vi "Test Serialization.vi"() -> ()   [LabVIEW 2014]
uses:
  reusable/PAS/Data/Main/PAS Data.lvclass
  <vilib>/NI/AQ Character Lineator/JSON Serializer/JSON Serializer.lvclass
  <vilib>/NI/AQ Character Lineator/Serialization Common/Serial Version.ctl
  reusable/PAS/Data/Cell/PAS Cell Data.lvclass
  <vilib>/NI/AQ Character Lineator/Formatter/Path Embedding.ctl
  reusable/CRDS/Data/Cell/CRDS Cell Data.lvclass
  reusable/CRDS/Data/Main/CRDS Data.lvclass
  reusable/CRDS/Cell/extParam Ctl.ctl
  reusable/CRDS/Cell/hkParam Ctl.ctl
  <vilib>/Platform/TimedLoop/XDataNode/XDataNode.xnode
  <vilib>/Platform/TimedLoop/XDataNode/nitl_modes.ctl
  <vilib>/Platform/TimedLoop/XDataNode/XDNodeRunTimeDep.lvlib
  <vilib>/Platform/TimedLoop/XDataNode/wakeup.ctl
  <vilib>/Platform/TimedLoop/XDataNode/timing_clust.ctl
panel:
  out "x-y":u32
  out "Global Start Time":i64
  in  "Boolean":bool
  in  "Stop Button":bool
  out "error out":errorcluster
  out "length":i32
  out "String":string
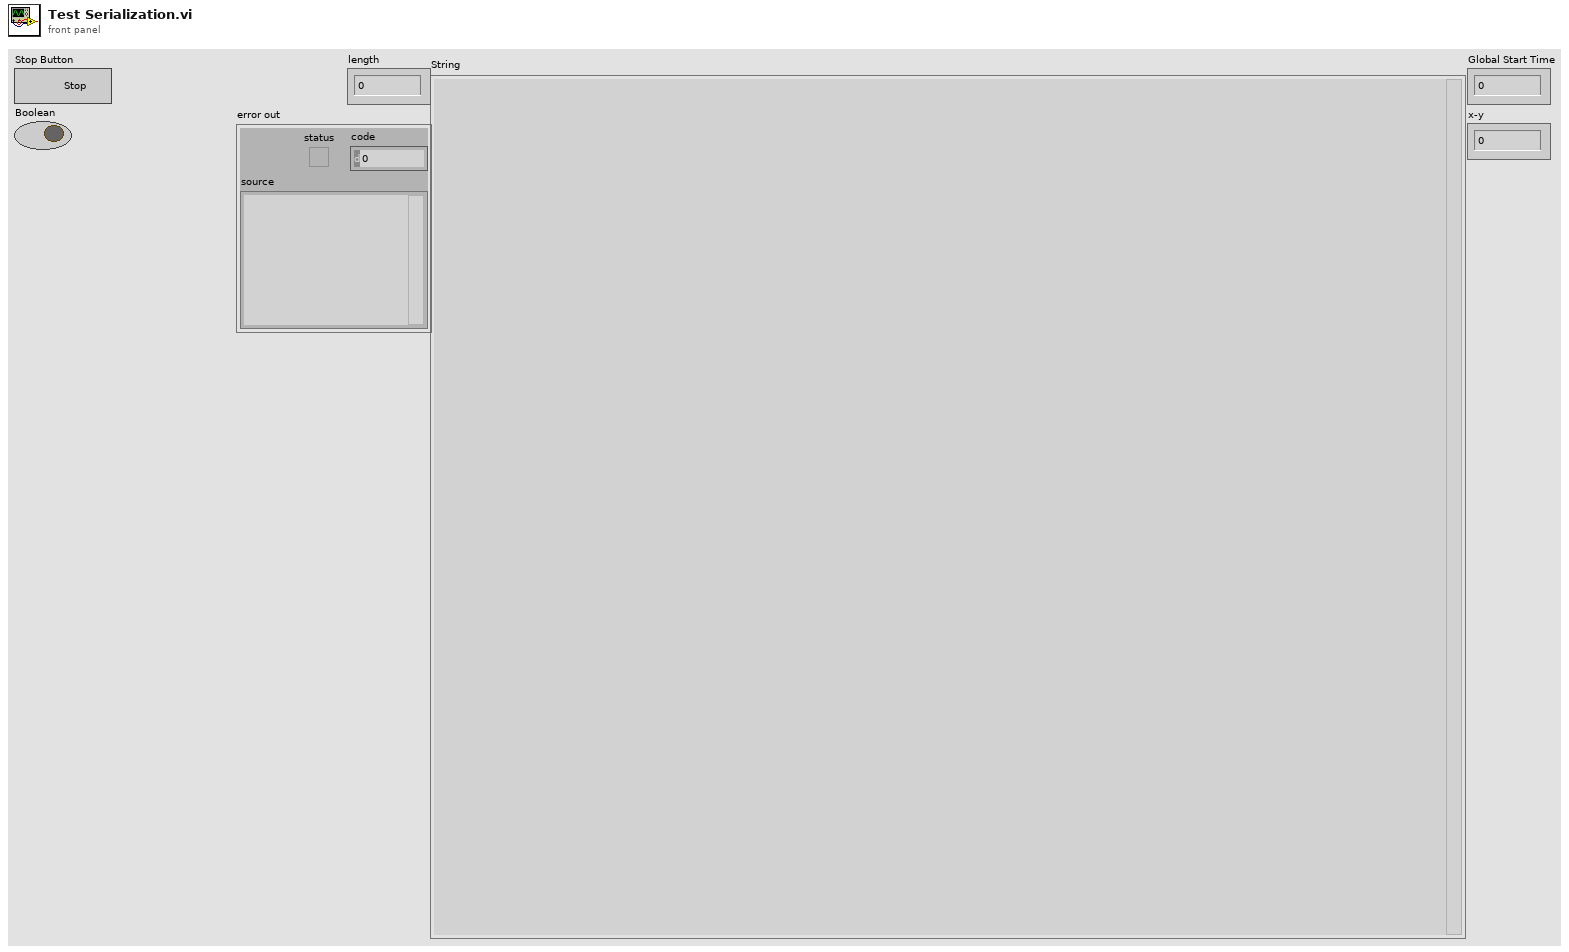
[diagram p1: front panel]
types:
  T1 = typedef "XDNodeRunTimeDep.lvlib/timing_clust.ctl" = cluster{"Expected End [f-1]":u64, "Actual End [f-1]":u64, "Finished Late? [f-1]":bool, "Expected End [i-1]":u64, "Actual End [i-1]":u64, "Finished Late? [i-1]":bool, "Expected Start [i]":u64, "Actual Start [i]":u64, "Expected Start [f]":u64, "Actual Start [f]":u64, "Source Name":string, "Structure Name":string, "Period":i64, "Deadline":i64, "Offset":i64, "Start":i64, "Priority":i32, "Timeout":i32, "Mode":T2, "Wakeup Reason":T3, "Error":errorcluster, "Source Type":string, "Secondary Source Type":string, "Global End Time":u64, "Global Start Time":u64, "Frame Duration":u64, "Iteration Duration":u64, "Assigned CPU":i32, "I/O Scan Engine Mode":u32}
  T2 = typedef "XDNodeRunTimeDep.lvlib/nitl_modes.ctl" = enum32{"No Change", "Process missed periods, maintain original phase", "Discard missed periods, maintain original phase", "Process missed periods, ignore original phase", "Discard missed periods, ignore original phase"}
  T3 = typedef "XDNodeRunTimeDep.lvlib/wakeup.ctl" = enum32{"Normal", "Aborted", "Asynchronous wakeup", "Timing source error", "Timed loop error", "Timeout"}
  T4 = typedef "Formatter.lvclass/Path Embedding.ctl" = enum16{"No paths embedded", "One path with each object", "All paths with each top object"}
  T5 = typedef "Serialization Common.lvlib/Serial Version.ctl" = cluster{"Major":u16, "Minor":u16, "Fix":u16, "Build":u16}
  T6 = typedef "CRDS Lib.lvlib/CRDS Cell Data.lvclass/hkParam Ctl.ctl" = cluster{"rhDilFac":sgl, "Q":sgl, "Tmean":sgl, "extDilFac":sgl, "rhCell":sgl, "P":sgl, "T":sgl}
  T7 = typedef "CRDS Lib.lvlib/CRDS Cell Data.lvclass/extParam Ctl.ctl" = cluster{"Tau":sgl, "Tau0cor":sgl, "ext":sgl, "extCorr":sgl, "stdevTau":sgl, "eTau":sgl, "taucorr":sgl, "Tau0":sgl, "max":sgl}
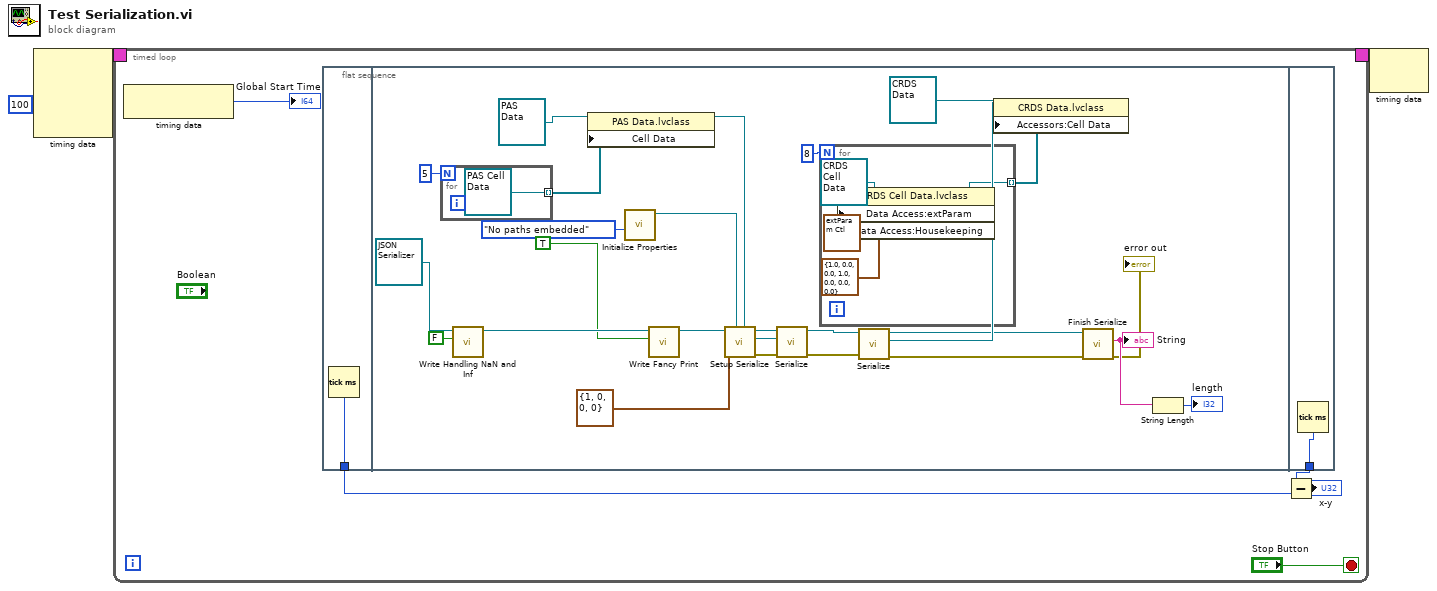
[diagram p0: block diagram]
diagram:
  n1 = node-c288(i64 100 ("Period")) -> (w3:T1)  [unwired: 3 in]
  n2 = timed-loop {
    timing: w3 -> [_]
    timing-out: [_] -> w2
    stop <- "Stop Button" stop-if-true
    n3 = node-c288() -> (→"Global Start Time":i64)  [unwired: 1 in]
    n4 = flat-sequence {
      tunnel: [w9] -> w5
      tunnel: [w40] -> w6
      frame #0 {
        n5 = Tick Count (ms)() -> (millisecond timer value=w9:u32)
      }
      frame #1 {
        n6 = for {
          N: 5 -> [_]
          tunnel: [refnum<class "PAS Cell Data.lvclass"> refnum ("Cell Data")] -> w26 mode=indexing
        }
        n7 = call <vilib>:"Write Handling NaN and Inf.vi"("Allow encoding NaN and Infinity?"=FALSE, "JSON Serializer in"=refnum<class "JSON Serializer.lvclass"> refnum ("TestSerializer.lvclass")) -> ("JSON Serializer out"=w33:refnum<class "JSON Serializer.lvclass">)  [unwired: 9 in]
        n8 = property class="PAS Data.lvclass"(reference=refnum<class "PAS Data.lvclass"> refnum ("PAS Data"), "Cell Data"=w26) -> (reference out=w10:refnum<class "PAS Data.lvclass">)  [unwired: 1 in, 1 out]
        n9 = call <vilib>:"Initialize Properties.vi"("Dynamic Path Behavior"=Path_Embedding."No paths embedded") -> ("Formatter out"=w24:refnum<class "Formatter.lvclass">)  [unwired: 10 in]
        n10 = call <vilib>:"Write Fancy Print.vi"("Fancy Print"=TRUE, "JSON Serializer in"=w33) -> ("JSON Serializer out"=w31:refnum<class "JSON Serializer.lvclass">)  [unwired: 9 in]
        n11 = call <vilib>:"Setup Serialize.vi"("Formatter (defaults)"=w24, "Serial Version"=T5 {"Major"=1, "Minor"=0, "Fix"=0, "Build"=0}, "Serializer in"=w31) -> ("error out"=w28:errorcluster, "Serializer out"=w29:refnum<class "JSON Serializer.lvclass">)  [unwired: 7 in]
        n12 = call-dynamic "Serialize.vi"("error in (no error)"=w28, "Serializable"=w10, "JSON Serializer in"=w29) -> ("error out"=w18:errorcluster, "JSON Serializer out"=w19:refnum<class "JSON Serializer.lvclass">)  [unwired: 7 in]
        n13 = for {
          N: 8 -> [_]
          tunnel: [w35] -> w15 mode=indexing
          n14 = property class="CRDS Cell Data.lvclass"(reference=refnum<class "CRDS Cell Data.lvclass"> refnum ("CRDS Cell"), "Data Access:extParam"=T7 {"Tau"=0.0, "Tau0cor"=0.0, "ext"=0.0, "extCorr"=0.0, "stdevTau"=0.0, "eTau"=0.0, "taucorr"=0.0, "Tau0"=0.0, "max"=0.0} ("extParam"), "Data Access:Housekeeping"=T6 {"rhDilFac"=1.0, "Q"=0.0, "Tmean"=0.0, "extDilFac"=1.0, "rhCell"=0.0, "P"=0.0, "T"=0.0} ("Housekeeping")) -> (reference out=w35:refnum<class "CRDS Cell Data.lvclass">)  [unwired: 1 in, 1 out]
        }
        n15 = property class="CRDS Data.lvclass"(reference=refnum<class "CRDS Data.lvclass"> refnum ("CRDS"), "Accessors:Cell Data"=w15) -> (reference out=w14:refnum<class "CRDS Data.lvclass">)  [unwired: 1 in, 1 out]
        n16 = call-dynamic "Serialize.vi"("error in (no error)"=w18, "Serializable"=w14, "JSON Serializer in"=w19) -> ("error out"=w12:errorcluster, "JSON Serializer out"=w13:refnum<class "JSON Serializer.lvclass">)  [unwired: 7 in]
        n17 = call <vilib>:"Finish Serialize.vi"("error in (no error)"=w12, "Serializer in"=w13) -> ("error out"=→"error out":errorcluster, "String"=w21:string)  [unwired: 6 in, 2 out]
        "String" <- w21
        n18 = String Length(string=w21) -> (length=→"length":i32)
      }
      frame #2 {
        n19 = Tick Count (ms)() -> (millisecond timer value=w40:u32)
      }
    }
    n20 = Subtract(x=w6, y=w5) -> (x-y=→"x-y":u32)
  }
  n21 = node-c288(w2) -> ()  [unwired: 1 out]
